vi "Start Message.vi"(8 "Error In":errorcluster, 9 "Retry Timeout ms (-1, use browser default)":i32=-1, 10 "Event Name (blank, message event)":string) -> (0 "Error Out":errorcluster, 3 "Message Out":string)   [LabVIEW 2014, in "i3-sse-server.lvlib"]
uses:
  i3-sse-server.lvlib
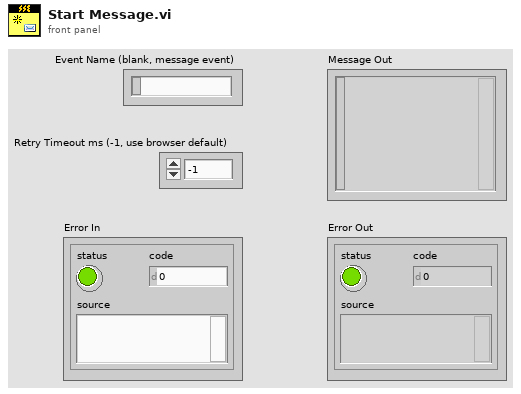
[diagram p1: front panel]
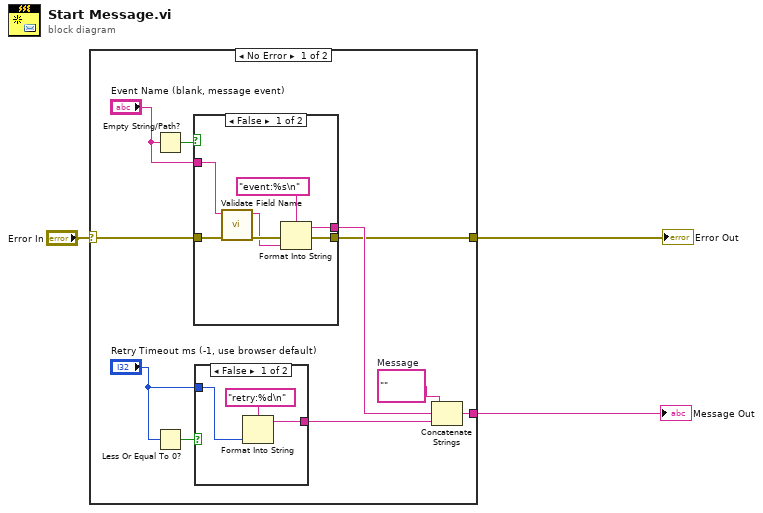
[diagram p0: block diagram]
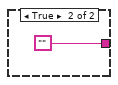
[diagram p2: hidden frame]
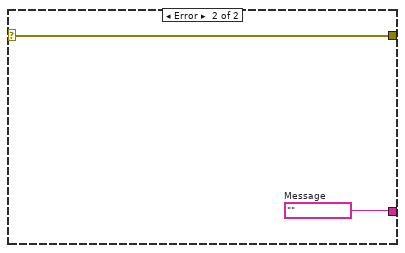
[diagram p4: hidden frame]
diagram:
  n1 = case shown="No Error" "Error In" {
    selector: "Error In" -> [w11 w28]
    tunnel: [w5 w28] -> w1
    tunnel: [w4 w27] -> w2
    frame No Error {
      w8 = ""  # Message
      n2 = Empty String/Path?(string/path="Event Name (blank, message event)") -> (empty?=w13:bool)
      n3 = Less Or Equal To 0?(x="Retry Timeout ms (-1, use browser default)") -> (x <= 0?=w10:bool)
      n4 = case shown="False" w13 {
        tunnel: "Event Name (blank, message event)" -> [w20 w25]
        tunnel: w11 -> [w22 w26]
        tunnel: [w23 w26] -> w5
        tunnel: [w24 w25] -> w7
        frame False {
          n5 = call "Validate Field Name.vi"("Error In"=w22, "Field Name In"=w20) -> ("Error Out"=w21:errorcluster, "Field Name Out"=w19:string)  [unwired: 8 in]
          n6 = Format Into String(format string="event:%s\n", error in=w21, w19) -> (resulting string=w24:string, error out=w23:errorcluster)  [unwired: 1 in]
        }
        frame True {
        }
      }
      n7 = case shown="False" w10 {
        tunnel: [w15 ""] -> w6
        tunnel: "Retry Timeout ms (-1, use browser default)" -> [w14 _]
        frame False {
          n8 = Format Into String(format string="retry:%d\n", w14) -> (resulting string=w15:string)  [unwired: 2 in, 1 out]
        }
        frame True {
        }
      }
      n9 = Concatenate Strings(w8, w7, w6) -> (w4:string)
    }
    frame Error {
      w27 = ""  # Message
    }
  }
  "Error Out" <- w1
  "Message Out" <- w2
